vi "Self Test.vi"(8 "error in":errorcluster, 11 "DAQ970 in":refnum<class "DAQ970.lvclass">) -> (0 "error out":errorcluster, 3 "DAQ970 out":refnum<class "DAQ970.lvclass">)   [LabVIEW 2019, in "DAQ970.lvlib" / "DAQ970.lvclass"]
doc: "This Override VI must be called by ancestor classes\nThis class reads error data and transmits it to the fault handler"
uses:
  Library/DAQ970.lvclass
  Library/DAQ970.lvclass/DAQ970.ctl
  builds/Instruments/Instruments.lvlibp/Library/Instruments.lvclass
  <instrlib>/Keysight DAQ970/Keysight DAQ970.lvlib
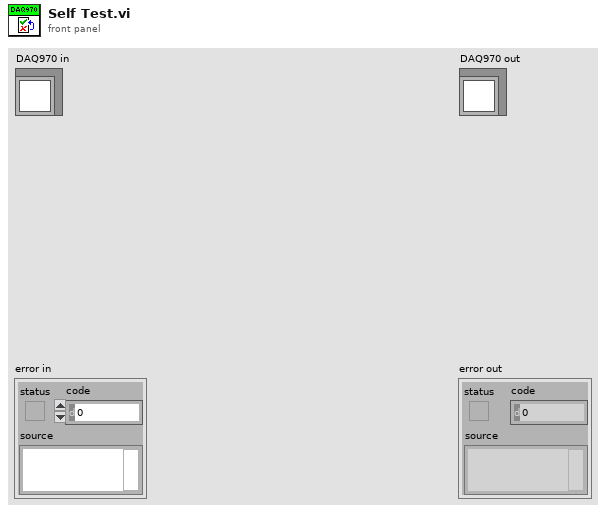
[diagram p1: front panel]
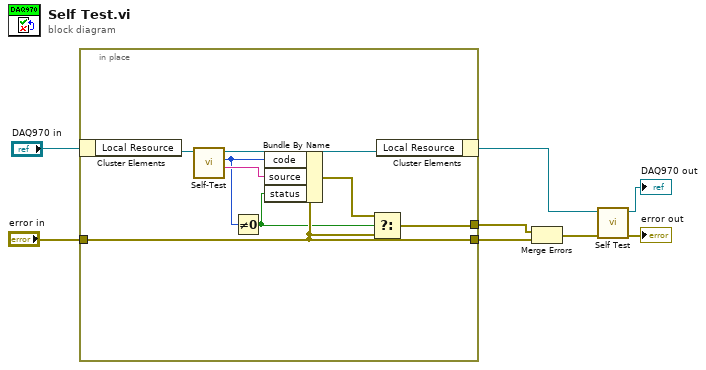
[diagram p0: block diagram]
diagram:
  n1 = in-place {
    in-place-border: "error in" -> [w13]
    in-place-border: [w13] -> w3
    in-place-border: [w14] -> w2
    n2 = in-place-cluster #1("DAQ970 in") -> ("Local Resource"=w16:refnum<k15>)
    n3 = call <instrlib>:"Self-Test.vi"("instrument handle"=w16) -> ("self-test message"=w11:string, "self test result"=w10:i16, "instrument handle out"=w15:refnum<k15>)  [unwired: 7 in, 1 out]
    n4 = Not Equal To 0?(x=w10) -> (x != 0?=w12:bool)
    n5 = Bundle By Name(cluster=w13, "code"=w10, "source"=w11, "status"=w12) -> (w9:errorcluster)
    n6 = Select(t=w9, s=w12, f=w13) -> (s? t:f=w14:errorcluster)
    n7 = in-place-cluster #1("Local Resource"=w15) -> (w4:refnum<class "DAQ970.lvclass">)
  }
  n8 = Merge Errors(w2, w3) -> (w1:errorcluster)
  n9 = call-parent "Self Test.vi"("error in"=w1, "Instruments in"=w4) -> ("error out"=→"error out":errorcluster, "Instruments out"=→"DAQ970 out":refnum<class "DAQ970.lvclass">)  [unwired: 8 in]
